vi "Write Funnel Settings.vi"(8 "error in (no error)":errorcluster, 10 "Funnel Settings.lvclass":refnum<class "Funnel Settings.lvclass">, 11 "Tool Funnel in":refnum<class "Tool Funnel.lvclass">) -> (0 "error out":errorcluster, 3 "Tool Funnel out":refnum<class "Tool Funnel.lvclass">)   [LabVIEW 2019, in "Tool Funnel.lvclass"]
uses:
  Tool Funnel.lvclass
  Settings/Funnel Settings/Funnel Settings.lvclass
  Tool Funnel.lvclass/Tool Funnel.ctl
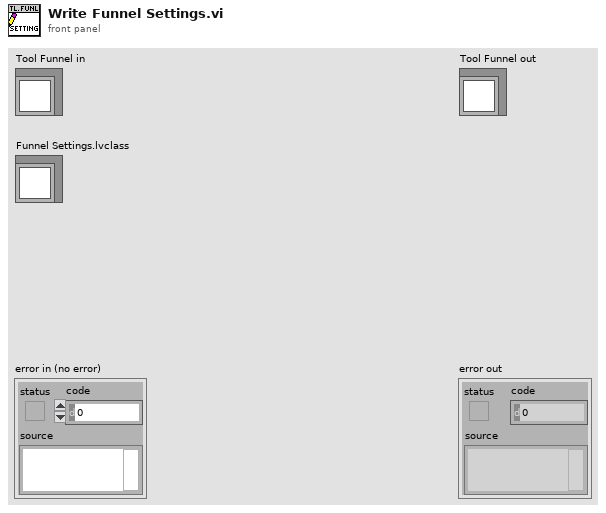
[diagram p1: front panel]
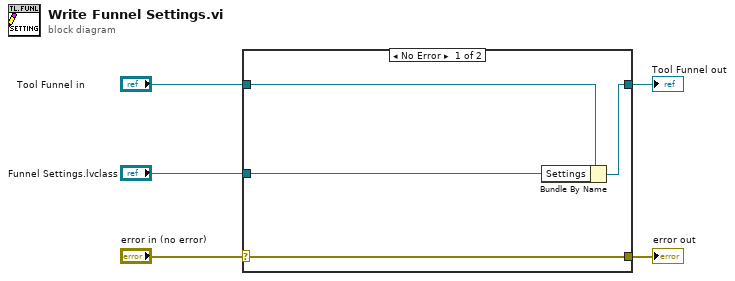
[diagram p0: block diagram]
diagram:
  n1 = case shown="No Error" "error in (no error)" {
    selector: "error in (no error)" -> [w9 w10]
    tunnel: [w9 w10] -> w4
    tunnel: [w7 w11] -> w2
    tunnel: "Tool Funnel in" -> [w8 w11]
    tunnel: "Funnel Settings.lvclass" -> [w6 _]
    frame No Error {
      n2 = Bundle By Name(cluster=w8, "Settings"=w6) -> (w7:refnum<class "Tool Funnel.lvclass">)
    }
    frame Error {
    }
  }
  "error out" <- w4
  "Tool Funnel out" <- w2
